vi "写入excel(参考灵敏度).vi"(7 "设置":string[](array[string])=["160", "10", "0.02", "0.02", "0.1", "10", "J5", "J6"], 8 "error in (no error)":errorcluster, 9 "被测幅值":dbl format="%.2p", 10 "参考幅值":dbl format="%.2p", 11 "NI_report输入":refnum<class "NI_report.lvclass">) -> (0 "error out":errorcluster, 3 "report out":refnum<class "NI_report.lvclass">)   [LabVIEW 2015]
uses:
  <vilib>/Utility/NIReport.llb/NI_report.lvclass
  <vilib>/addons/_office/_exclsub.llb/font.ctl
  Global.vi
  <vilib>/Utility/NIReport.llb/Excel/NI_Excel.lvclass
  <vilib>/addons/_office/NI_ReportGenerationToolkit.lvlib
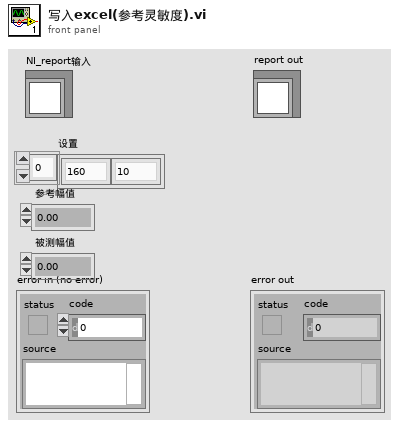
[diagram p1: front panel]
types:
  T1 = typedef "NI_ReportGenerationToolkit.lvlib/font.ctl" = cluster{"font name":string, "font size":dbl, "bold":u16, "italic":u16, "underline":u16, "strike through":u16, "font color":u32}
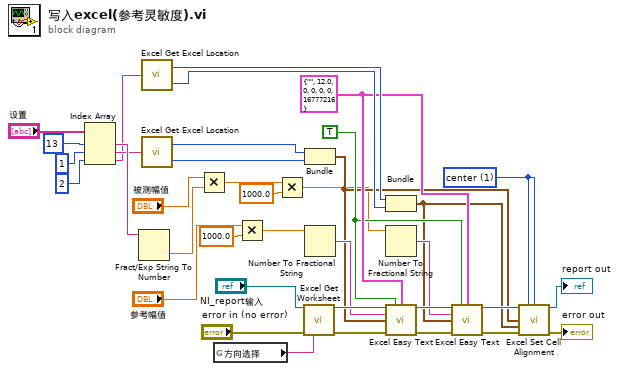
[diagram p0: block diagram]
diagram:
  w7 = 1 items=["top", "center", "bottom"] ("vertical alignment (top)")
  w14 = TRUE ("border? (F)")
  w15 = T1 {"font name"="", "font size"=12.0, "bold"=0, "italic"=0, "underline"=0, "strike through"=0, "font color"=16777216} ("font")
  n1 = Index Array(array="设置", index #1=13 ("索引"), index #2=1 ("索引 (行)"), index #3=2 ("索引")) -> (element #1=w27:string, element #2=w24:string, element #3=w18:string)
  n2 = Fract/Exp String To Number(string=w27) -> (number=w26:dbl)  [unwired: 3 in, 1 out]
  n3 = call <vilib>:"Excel Get Excel Location.vi"("cell's name"=w18) -> ("row"=w17:i32, "column"=w16:i32)
  n4 = call <vilib>:"Excel Get Excel Location.vi"("cell's name"=w24) -> ("row"=w23:i32, "column"=w22:i32)
  n5 = Multiply(x="被测幅值", y=w26) -> (x*y=w6:dbl)
  n6 = global read "Global.vi" "方向选择"() -> (w33:string)
  n7 = Multiply(x="参考幅值", y=1000.0) -> (x*y=w1:dbl)
  n8 = Multiply(x=w6, y=1000.0) -> (x*y=w4:dbl)
  n9 = call <vilib>:"Excel Get Worksheet.vi"("report in"="NI_report输入", "error in (no error)"="error in (no error)", "name (\"\")"=w33) -> ("report out"=w35:refnum<class "NI_report.lvclass">, "error out"=w34:errorcluster)  [unwired: 11 in]
  n10 = Bundle("row"=w23, "column"=w22) -> (w9:cluster{"row":i32, "column":i32})  [unwired: 1 in]
  n11 = Number To Fractional String(number=w1) -> (F-format string=w25:string)  [unwired: 3 in]
  n12 = Bundle("row"=w17, "column"=w16) -> (w8:cluster{"row":i32, "column":i32})  [unwired: 1 in]
  n13 = Number To Fractional String(number=w4) -> (F-format string=w19:string)  [unwired: 3 in]
  n14 = call <vilib>:"Excel Easy Text.vi"("report in"=w35, "border? (F)"=w14, "font"=w15, "text"=w25, "start (-1, -1)"=w9, "error in (no error)"=w34) -> ("report out"=w21:refnum<class "NI_report.lvclass">, "error out"=w20:errorcluster)  [unwired: 5 in, 3 out]
  n15 = call <vilib>:"Excel Easy Text.vi"("report in"=w21, "border? (F)"=w14, "font"=w15, "text"=w19, "start (-1, -1)"=w8, "error in (no error)"=w20) -> ("report out"=w13:refnum<class "NI_report.lvclass">, "error out"=w12:errorcluster)  [unwired: 5 in, 3 out]
  n16 = call <vilib>:"Excel Set Cell Alignment.vi"("report in"=w13, "vertical alignment (top)"=w7, "horizontal alignment (left)"=w7, "start (-1, -1)"=w9, "end (-1, -1)"=w8, "error in (no error)"=w12) -> ("report out"=→"report out":refnum<class "NI_report.lvclass">, "error out"=→"error out":errorcluster)  [unwired: 8 in]
